vi "TCP Initialize Connection Manager (By Reference).vi"(8 "error in (no error)":errorcluster) -> (0 "error out":errorcluster, 3 "connection manager ref out":T1)   [LabVIEW 2010, in "NI STM.lvlib"]
uses:
  TCP Connection Manager Reference.ctl
  TCP Connection Manager State Variables.ctl
  TCP/TCP Connection Info.ctl
  SubVIs/MetaDataElement.ctl
  TCP Connection Properties.ctl
  NI STM.lvlib
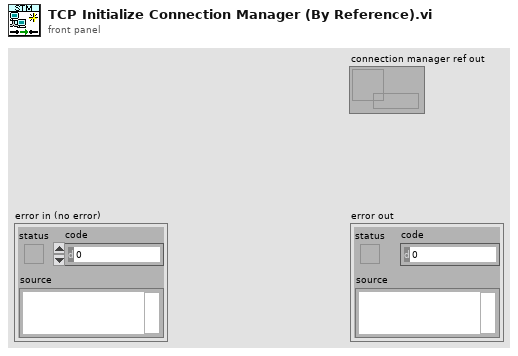
[diagram p1: front panel]
types:
  T1 = typedef "NI STM.lvlib/TCP Connection Manager Reference.ctl" = refnum<data-value>
  T2 = typedef "NI STM.lvlib/TCP Connection Manager State Variables.ctl" = cluster{"Connections":T3[], "Properties":T5[]}
  T3 = typedef "NI STM.lvlib/TCP Connection Info.ctl" = cluster{"connection ID":refnum<k5>, "meta data":T4[]}
  T4 = typedef "NI STM.lvlib/MetaDataElement.ctl" = string
  T5 = typedef "NI STM.lvlib/TCP Connection Properties.ctl" = cluster{"Name":string, "Address":string, "Custom":string}
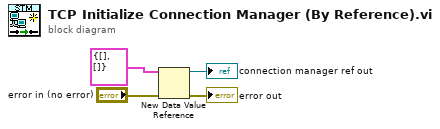
[diagram p0: block diagram]
diagram:
  n1 = New Data Value Reference(data value=T2 {"Connections"=[], "Properties"=[]}, error in="error in (no error)") -> (data value reference=→"connection manager ref out":refnum<data-value>, error out=→"error out":errorcluster)
